vi "Write Status.vi"(8 "Error In":errorcluster, 10 "Attributes In":refnum<class "SFTP Attributes.lvclass">, 11 "SFTP File In":refnum<class "SFTP File.lvclass">) -> (0 "Error Out":errorcluster, 2 "Attributes Out":refnum<class "SFTP Attributes.lvclass">, 3 "SFTP File Out":refnum<class "SFTP File.lvclass">)   [LabVIEW 2018, in "Toolkit.lvlib" / "SFTP File.lvclass"]
uses:
  SFTP File.lvclass
  SFTP Attributes/SFTP Attributes.lvclass
  SFTP File.lvclass/SFTP File.ctl
  SFTP Attributes/SFTP Attributes.lvclass/SFTP Attributes.ctl
  SFTP/SFTP.lvclass/SFTP.ctl
  Toolkit.lvlib
  SFTP/SFTP.lvclass
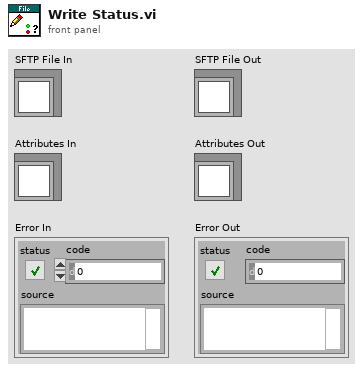
[diagram p1: front panel]
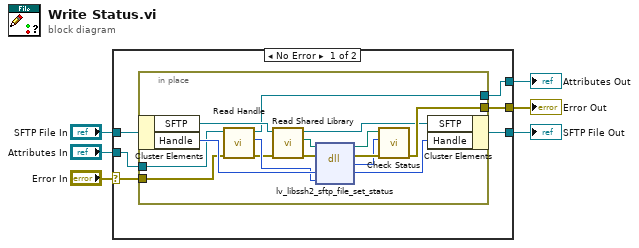
[diagram p0: block diagram]
diagram:
  n1 = case shown="No Error" "Error In" {
    selector: "Error In" -> [w11 w29]
    tunnel: "SFTP File In" -> [w12 w30]
    tunnel: [w10 w30] -> w3
    tunnel: [w9 w29] -> w4
    tunnel: "Attributes In" -> [w8 w28]
    tunnel: [w7 w28] -> w1
    frame No Error {
      n2 = in-place {
        in-place-border: w11 -> [w15]
        in-place-border: [w22] -> w9
        in-place-border: w8 -> [w17]
        in-place-border: [w13] -> w7
        n3 = in-place-cluster #1(w12) -> ("SFTP"=w20:refnum<class "SFTP.lvclass">, "Handle"=w27:u64)
        n4 = call "Read Handle.vi"("Error In"=w15, "SFTP Attributes In"=w17) -> ("Error Out"=w14:errorcluster, "Handle"=w16:u64, "SFTP Attributes Out"=w13:refnum<class "SFTP Attributes.lvclass">)  [unwired: 7 in]
        n5 = call "Read Shared Library.vi"("Error In"=w14, "SFTP In"=w20) -> ("Erorr Out"=w21:errorcluster, "lv-libssh2 Shared Library"=w18:path, "SFTP Out"=w19:refnum<class "SFTP.lvclass">)  [unwired: 7 in]
        n6 = dll-call lib="libssh2lv.*" fn="lv_libssh2_sftp_file_set_status"(path in=w18, error in=w21, "handle"=w27, "attributes"=w16) -> (path out=w24:path, error out=w25:errorcluster, "status"=w23:i32, "handle"=w26:u64)  [unwired: 2 in]
        n7 = call "Check Status.vi"("Error In"=w25, "Status"=w23, "lv-libssh2 Shared Library In"=w24) -> ("Error Out"=w22:errorcluster)  [unwired: 7 in, 1 out]
        n8 = in-place-cluster #1("SFTP"=w19, "Handle"=w26) -> (w10:refnum<class "SFTP File.lvclass">)
      }
    }
    frame Error {
    }
  }
  "Error Out" <- w4
  "SFTP File Out" <- w3
  "Attributes Out" <- w1
